vi "十六进制字符串到数值.vi"(10 "字符串":string) -> (2 "数值":string, 3 "数值":i32)   [LabVIEW 2013]
panel:
  out "x*y":u32
  out "元素":u8
  out "字符串 3":string
  out "无符号字节数组":u8[](array[numeric])
  out "长度":i32
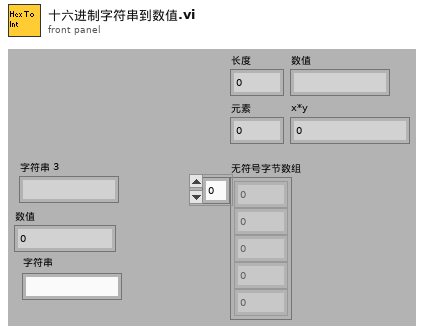
[diagram p1: front panel]
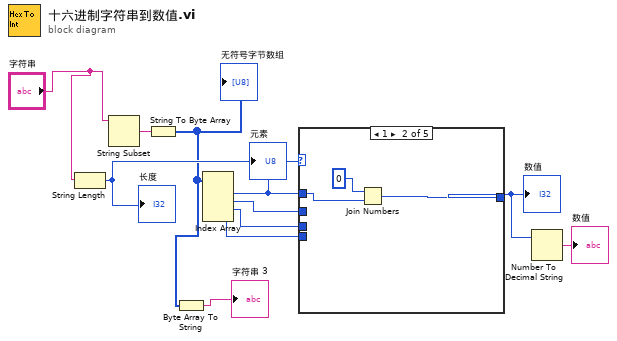
[diagram p0: block diagram]
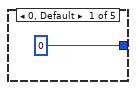
[diagram p2: hidden frame]
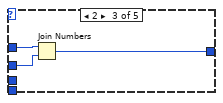
[diagram p3: hidden frame]
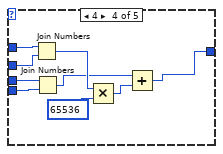
[diagram p4: hidden frame]
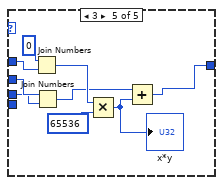
[diagram p5: hidden frame]
diagram:
  n1 = String Length(string="字符串") -> (length=w7:i32)
  "长度" <- w7
  n2 = String Subset(string="字符串") -> (substring=w11:string)  [unwired: 2 out]
  n3 = String To Byte Array(string=w11) -> (unsigned byte array=w3:u8[])
  "无符号字节数组" <- w3
  n4 = Byte Array To String(unsigned byte array=w3) -> (string=→"字符串 3":string)
  n5 = Index Array(array=w3) -> (element #1=w10:u8, element #2=w9:u8, element #3=w6:u8, element #4=w5:u8)  [unwired: 4 in]
  "元素" <- w10
  n6 = case shown="1" w7 {
    tunnel: w10 -> [_ w14 w18 w27 w30]
    tunnel: w9 -> [_ _ w17 w26 w29]
    tunnel: [u16 0 w15 w16 w22 w35] -> w2
    tunnel: w6 -> [_ _ _ w25 w28]
    tunnel: w5 -> [_ _ _ w24 _]
    frame 0, Default {
    }
    frame 1 {
      n7 = Join Numbers(hi=u8 0, lo=w14) -> ((hi.lo)=w15:u16)
    }
    frame 2 {
      n8 = Join Numbers(hi=w18, lo=w17) -> ((hi.lo)=w16:u16)
    }
    frame 4 {
      n9 = Join Numbers(hi=w27, lo=w26) -> ((hi.lo)=w20:u16)
      n10 = Join Numbers(hi=w25, lo=w24) -> ((hi.lo)=w19:u16)
      n11 = Multiply(x=w20, y=u32 65536) -> (x*y=w21:u32)
      n12 = Add(x=w19, y=w21) -> (x+y=w22:u32)
    }
    frame 3 {
      n13 = Join Numbers(hi=u8 0, lo=w30) -> ((hi.lo)=w33:u16)
      n14 = Join Numbers(hi=w29, lo=w28) -> ((hi.lo)=w32:u16)
      n15 = Multiply(x=w33, y=u32 65536) -> (x*y=w34:u32)
      "x*y" <- w34
      n16 = Add(x=w32, y=w34) -> (x+y=w35:u32)
    }
  }
  "数值" <- w2
  n17 = Number To Decimal String(number=w2) -> (decimal integer string=→"数值":string)  [unwired: 1 out]
